vi "_DServerRequestDataToDoubleScalar.vi"(0 "client request":T1={"Request Id"=0, "Source Id"=0, "Request Type"=enum."UNKNOWN_REQUEST", "Device Class Name"="unspecified_class_name", "Device Name"="unspecified/device/name", "Cmd or Attr Name"="unspecified_cmd_or_attr_name", "Client Request Data"={"write attribute value"={"dimx"=0, "dimy"=0, "data"=[], "data_type"=enum."UNKNOWN_DATA_TYPE"}, "exec. command argin"={"num data"=[], "str data"=[]}}}) -> (1 "attribute value":dbl, 2 "client request":T1={"Request Id"=0, "Source Id"=0, "Request Type"=enum."UNKNOWN_REQUEST", "Device Class Name"="unspecified_class_name", "Device Name"="unspecified/device/name", "Cmd or Attr Name"="unspecified_cmd_or_attr_name", "Client Request Data"={"write attribute value"={"dimx"=0, "dimy"=0, "data"=[], "data_type"=enum."UNKNOWN_DATA_TYPE"}, "exec. command argin"={"num data"=[], "str data"=[]}}})   [LabVIEW 2014, in "tango.lvlib"]
uses:
  tango.lvlib
  Typedefs/_DServerClientRequest.ctl
  Typedefs/_DServerClientRequestType.ctl
  Typedefs/_DServerClientRequestData.ctl
  Typedefs/_GenericDataBuffer.ctl
  Typedefs/_DataType.ctl
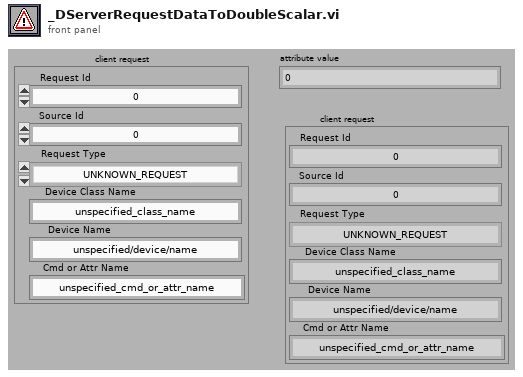
[diagram p1: front panel]
types:
  T1 = typedef "tango.lvlib/_DServerClientRequest.ctl" = cluster{"Request Id":u32, "Source Id":u32, "Request Type":T2, "Device Class Name":string, "Device Name":string, "Cmd or Attr Name":string, "Client Request Data":T3}
  T2 = typedef "tango.lvlib/_DServerClientRequestType.ctl" = enum16{"EXEC_CMD", "READ_ATTR", "WRITE_ATTR", "UNKNOWN_REQUEST"}
  T3 = typedef "tango.lvlib/_DServerClientRequestData.ctl" = cluster{"write attribute value":T4, "exec. command argin":cluster{"num data":u8[], "str data":string[]}}
  T4 = typedef "tango.lvlib/_GenericDataBuffer.ctl" = cluster{"dimx":u32, "dimy":u32, "data":u8[], "data_type":T5}
  T5 = typedef "tango.lvlib/_DataType.ctl" = enum16{"STATE_SCA", "STATE_SPE", "STATE_IMG", "STRING_SCA", "STRING_SPE", "STRING_IMG", "BOOL_SCA", "BOOL_SPE", "BOOL_IMG", "UCHAR_SCA", "UCHAR_SPE", "UCHAR_IMG", "SHORT_SCA", "SHORT_SPE", "SHORT_IMG", "USHORT_SCA", "USHORT_SPE", "USHORT_IMG", "LONG_SCA", "LONG_SPE", "LONG_IMG", "ULONG_SCA", "ULONG_SPE", "ULONG_IMG", "LONG64_SCA", "LONG64_SPE", "LONG64_IMG", "ULONG64_SCA", "ULONG64_SPE", "ULONG64_IMG", "FLOAT_SCA", "FLOAT_SPE", "FLOAT_IMG", "DOUBLE_SCA", "DOUBLE_SPE", "DOUBLE_IMG", "SCA_ENCODED", "SPE_ENCODED", "IMG_ENCODED", "UNKNOWN_DATA_TYPE"}
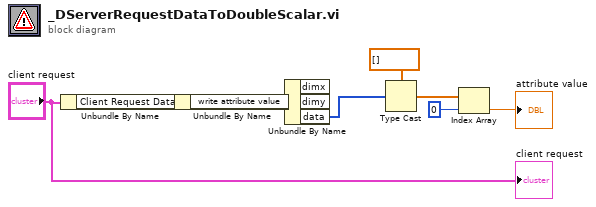
[diagram p0: block diagram]
diagram:
  n1 = Unbundle By Name("client request") -> ("Client Request Data"=w4:T3)
  n2 = Unbundle By Name(w4) -> ("write attribute value"=w3:T4)
  n3 = Unbundle By Name(w3) -> ("data"=w2:u8[])  [unwired: 2 out]
  n4 = Type Cast(type=dbl[] [], x=w2) -> (*(type *) &x=w6:dbl[])
  n5 = Index Array(array=w6, index=0 ("indice")) -> (element=→"attribute value":dbl)
  "client request" <- "client request"
